vi "Is Log All.vi"(7 "Action":T1, 11 "Log All?":bool) -> (4 "Log All?":bool)   [LabVIEW 2016, in "Stream Error.lvlib" / "Error Interface.lvclass"]
doc: "--\nCopyright © 2017 Composed SystemsI All rights reserved.\n\nAuthor: Jon McBee <jon.mcbee@composed.io>\n\nThis library is provided \"AS IS\" ,WITHOUT WARRANTIES OR\nCONDITIONS OF ANY KIND, either express or implied.\n\nComposed Systems -- composed.io\n\nStream 0.0.1.1\nJon McBee - Composed Systems\nCopyright (c) 2017, Composed Systems"
uses:
  <userlib>/Composed Systems/Stream/Error/Classes/Error Interface/Error Interface.lvclass
  <userlib>/Composed Systems/Stream/Error/Classes/Error Interface/Log Action States.ctl
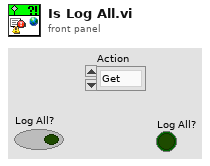
[diagram p1: front panel]
types:
  T1 = typedef "Stream Error.lvlib/Error Interface.lvclass/Log Action States.ctl" = enum16{"Get", "Set"}
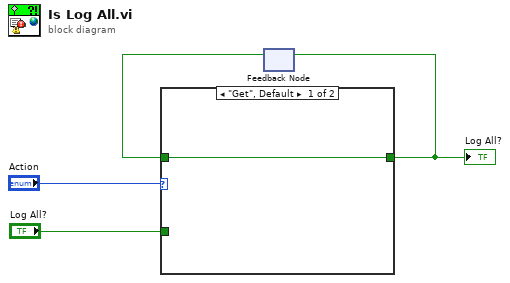
[diagram p0: block diagram]
diagram:
  n1 = feedback #1() -> (w1:bool)  [unwired: 1 in]
  n2 = case shown="\"Get\", Default" "Action" {
    tunnel: "Log All?" -> [_ w6]
    tunnel: w1 -> [w5 _]
    tunnel: [w5 w6] -> w2
    frame "Get", Default {
    }
    frame "Set" {
    }
  }
  "Log All?" <- w2
  n3 = feedback-in #1(w2) -> ()
